vi "Process.vi"(8 "error in (no error)":errorcluster, 9 "Sensor Groups (false)":bool, 10 "Pound in":refnum<class "Pound.lvclass">, 11 "Qbus in":refnum<class "Qbus.lvclass">) -> (0 "error out":errorcluster)   [LabVIEW 2017, in "OPCUAClient.lvlib"]
uses:
  <vilib>/addons/InsightCM/Devices/Shared/Common/OPCUAClient/OPCUAClient.lvlib
  <vilib>/addons/Qbus/Qbus.lvclass
  <vilib>/NI/Software Watchdog/Pound/Pound.lvclass
  <vilib>/addons/InsightCM/Devices/Shared/Common/OPCUAClient/controls/config.ctl
  <vilib>/OPCUA/controls/OPC UA Client Refnum.ctl
  <vilib>/addons/InsightCM/Devices/Shared/Common/OPCUAClient/controls/group.ctl
  <vilib>/addons/InsightCM/Devices/Shared/Common/OPCUAClient/controls/tag.ctl
  <vilib>/OPCUA/controls/Time Out.ctl
  <vilib>/addons/TraceLogger/TraceLogger.lvlib
  <vilib>/NI/Software Watchdog/Watchdog/Watchdog.lvclass
  <vilib>/addons/InsightCM/Utilities/GlobalConfiguration/GlobalConfiguration.lvlib
  <vilib>/addons/InsightCM/Devices/Shared/Common/DataEventCreator/DataEventCreator.lvlib
  <vilib>/OPCUA/NI OPC UA Client.lvlib
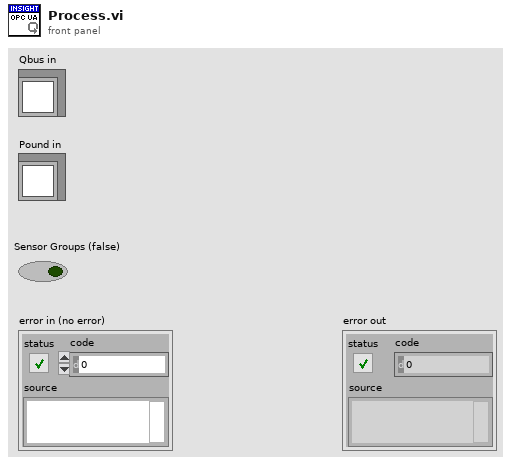
[diagram p1: front panel]
types:
  T1 = typedef "OPCUAClient.lvlib/config.ctl" = cluster{"OPC UA client refnum":T2, "Endpoint URL":string, "Client Certificate":path, "Server Certificate":path, "security policy":cluster{"message mode":enum16{"None", "Sign", "Sign and Encrypt"}, "security":enum16{"Basic256", "Basic128Rsa15"}}, "username/password":cluster{"username":string, "password":string}, "groups":T3[], "Read Interval (sec)":dbl, "Read Timeout (sec)":dbl, "Reconnect Interval (sec)":dbl, "Connection Timeout (sec)":dbl}
  T2 = typedef "OPC UA Client Refnum.ctl" = refnum<k21>
  T3 = typedef "OPCUAClient.lvlib/group.ctl" = cluster{"name":string, "Tags":T4[]}
  T4 = typedef "OPCUAClient.lvlib/tag.ctl" = cluster{"Id":string, "Tag":string, "Slope":dbl, "Offset":dbl}
  T5 = typedef "Time Out.ctl" = u32
  T6 = typedef "DataEventCreator.lvlib/RegisterTrendPoints.ctl" = cluster{"DataGroup":string, "Trends":T7[]}
  T7 = typedef "DataEventCreator.lvlib/Registry_Trend.ctl" = cluster{"TrendPointId":string, "DataSetName":string, "HighRate":bool, "Always Send":bool}
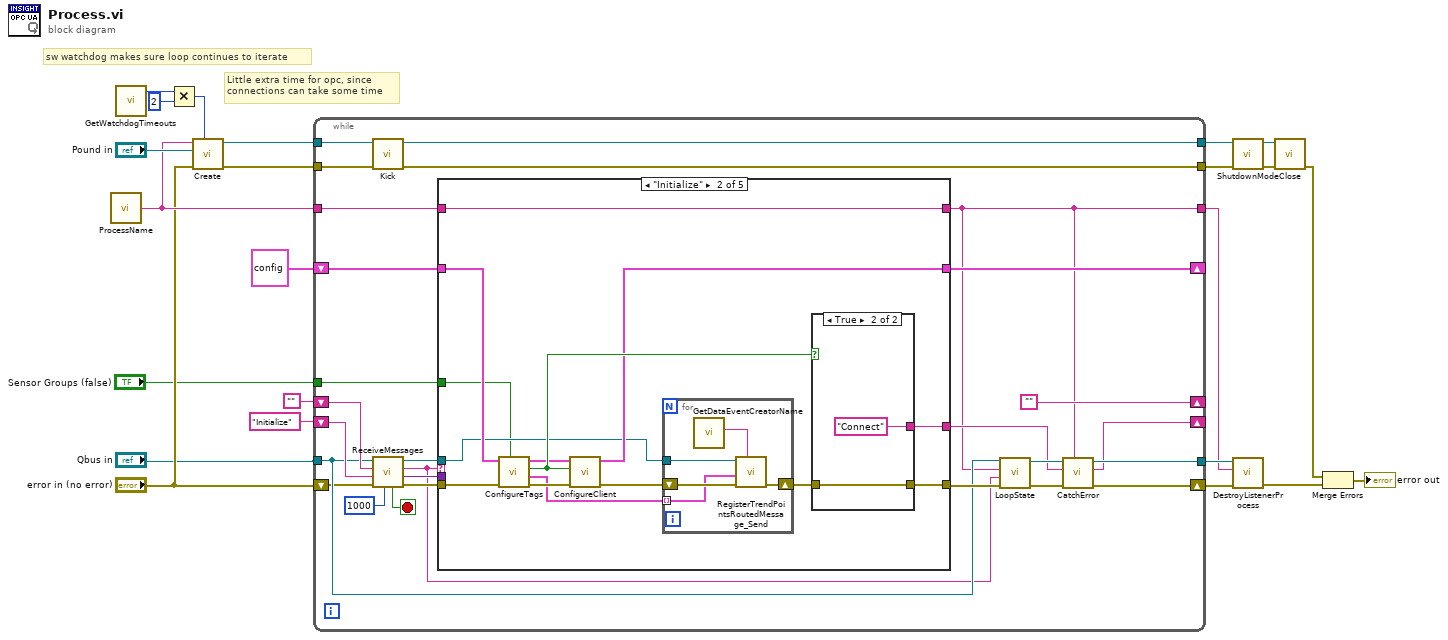
[diagram p0: block diagram]
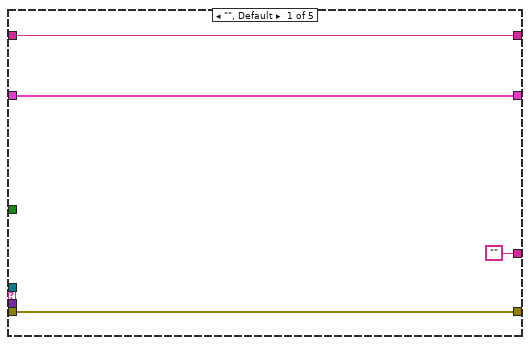
[diagram p2: hidden frame]
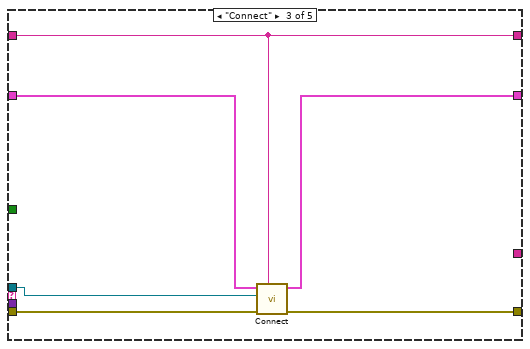
[diagram p4: hidden frame]
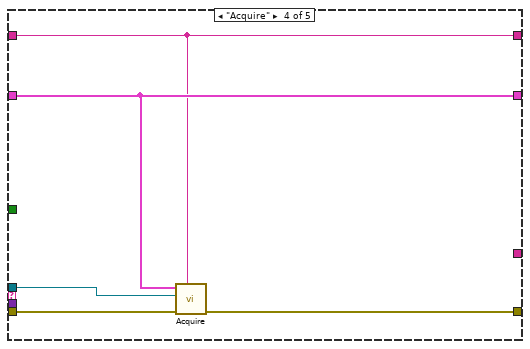
[diagram p5: hidden frame]
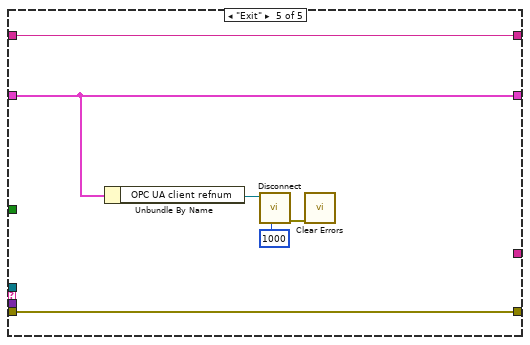
[diagram p6: hidden frame]
diagram:
  # "Little extra time for opc, since \nconnections can take some time"
  # "sw watchdog makes sure loop continues to iterate"
  n1 = call <vilib>:"ProcessName.vi"() -> ("process name"=w8:string)  [unwired: 5 in]
  n2 = call <vilib>:"GetWatchdogTimeouts.vi"() -> ("software timeout"=w3:u32)  [unwired: 10 in, 1 out]
  n3 = Multiply(x=w3, y=u32 2) -> (x*y=w1:u32)
  n4 = call <vilib>:"Create.vi"("Execution Timeout (ms)"=w1, "error in (no error)"="error in (no error)", "Pound"="Pound in", "Name"=w8) -> ("error out"=w13:errorcluster, "Watchdog"=w18:refnum<data-value>)  [unwired: 6 in]
  n5 = while {
    shift-right: [""] -> _
    shift-left: "" -> [w49]
    tunnel: "Qbus in" -> [w37]
    tunnel: w8 -> [w27]
    tunnel: [w40] -> w21
    tunnel: [w25] -> w20
    shift-right: [w39] -> _
    shift-left: "Initialize" -> [w44]
    shift-right: [w42] -> _
    shift-left: T1 {"OPC UA client refnum"="", "Endpoint URL"="", "Client Certificate"=path "", "Server Certificate"=path "", "security policy"={"message mode"=enum."None", "security"=enum."Basic256"}, "username/password"={"username"="", "password"=""}, "groups"=[], "Read Interval (sec)"=0.0, "Read Timeout (sec)"=0.0, "Reconnect Interval (sec)"=0.0, "Connection Timeout (sec)"=0.0} ("config") -> [w43]
    tunnel: w18 -> [w36]
    tunnel: [w35] -> w15
    tunnel: w13 -> [w34]
    tunnel: [w32] -> w12
    shift-right: [w41] -> w22
    shift-left: "error in (no error)" -> [w33]
    tunnel: "Sensor Groups (false)" -> [w24]
    stop <- w50 stop-if-true
    n6 = call <vilib>:"Kick.vi"("error in (no error)"=w34, "Watchdog"=w36) -> ("error out"=w32:errorcluster, "Watchdog"=w35:refnum<data-value>)  [unwired: 8 in]
    n7 = call <vilib>:"ReceiveMessages.vi"("Timeout(1000)"=1000 ("milliseconds to wait"), "error in (no error)"=w33, "priority action"=w44, "default action"=w49, "Qbus in"=w37) -> ("error out"=w48:errorcluster, "message value"=w45:variant, "action"=w31:string, "Qbus out"=w46:refnum<class "Qbus.lvclass">, "exit"=w50:bool)  [unwired: 2 in]
    n8 = case shown="\"Initialize\"" w31 {
      tunnel: w48 -> [w51 w64 w82 w86 w93]
      tunnel: w46 -> [_ w57 w78 w84 _]
      tunnel: [w51 w67 w77 w87 w93] -> w38
      tunnel: w45 -> [_ _ _ _ _]
      tunnel: w43 -> [w54 w65 w81 w85 w91]
      tunnel: [w54 w60 w80 w85 w91] -> w42
      tunnel: [w53 w68 w79 w83 w92] -> w25
      tunnel: w27 -> [w53 w68 w79 w83 w92]
      tunnel: ["" w66 _ _ _] -> w26
      tunnel: w24 -> [_ w55 _ _ _]
      frame "", Default {
      }
      frame "Initialize" {
        n9 = call <vilib>:"ConfigureTags.vi"("Sensor Groups (false)"=w55, "error in (no error)"=w64, "config in"=w65) -> ("error out"=w63:errorcluster, "Registrations"=w56:T6[], "Start OPC Client"=w62:bool, "config out"=w61:T1)  [unwired: 5 in]
        n10 = call <vilib>:"ConfigureClient.vi"("error in (no error)"=w63, "Start OPC Client"=w62, "config in"=w61) -> ("error out"=w59:errorcluster, "config out"=w60:T1)  [unwired: 7 in]
        n11 = for {
          shift-right: [w72] -> w58
          shift-left: w59 -> [w73]
          tunnel: w57 -> [w71]
          tunnel: w56 -> [w70] mode=indexing
          n12 = call <vilib>:"GetDataEventCreatorName.vi"() -> ("data event creator"=w69:string)  [unwired: 9 in, 2 out]
          n13 = call <vilib>:"RegisterTrendPointsRoutedMessage_Send.vi"("data event creator process name"=w69, "error in (no error)"=w73, "register trend"=w70, "Qbus in"=w71) -> ("error out"=w72:errorcluster)  [unwired: 6 in, 1 out]
        }
        n14 = case shown="True" w62 {
          tunnel: [w74 w76] -> w67
          tunnel: w58 -> [w74 w76]
          tunnel: [_ "Connect"] -> w66
          frame False {
          }
          frame True {
          }
        }
      }
      frame "Connect" {
        n15 = call <vilib>:"Connect.vi"("Process Name"=w79, "error in (no error)"=w82, "Qbus"=w78, "config"=w81) -> ("error out"=w77:errorcluster, "config out"=w80:T1)  [unwired: 5 in, 1 out]
      }
      frame "Acquire" {
        n16 = call <vilib>:"Acquire.vi"("Module Name"=w83, "error in (no error)"=w86, "Qbus in"=w84, "config"=w85) -> ("error out"=w87:errorcluster)  [unwired: 7 in]
      }
      frame "Exit" {
        n17 = Unbundle By Name(w91) -> ("OPC UA client refnum"=w90:T2)
        n18 = call <vilib>:"Disconnect.vi"("timeout (5000 ms)"=T5 1000, "OPC UA client refnum in"=w90) -> ("error out"=w89:errorcluster)  [unwired: 9 in]
        n19 = call <vilib>:"Clear Errors.vi"("error in (no error)"=w89) -> ()  [unwired: 5 in, 2 out]
      }
    }
    n20 = call <vilib>:"LoopState.vi"("error in (no error)"=w38, "loop action"=w31, "process name"=w25, "Qbus in"=w37) -> ("error out"=w29:errorcluster, "Qbus out"=w28:refnum<class "Qbus.lvclass">)  [unwired: 6 in]
    n21 = call <vilib>:"CatchError.vi"("source"=w25, "error in (no error)"=w29, "next action in"=w26, "Qbus in"=w28) -> ("error out"=w41:errorcluster, "next action out"=w39:string, "Qbus out"=w40:refnum<class "Qbus.lvclass">)  [unwired: 5 in]
  }
  n22 = call <vilib>:"ShutdownMode.vi"("error in (no error)"=w12, "Watchdog"=w15) -> ("error out"=w14:errorcluster, "Watchdog"=w16:refnum<data-value>)  [unwired: 8 in]
  n23 = call <vilib>:"DestroyListenerProcess.vi"("error in (no error)"=w22, "process name"=w20, "Qbus in"=w21) -> ("error in (no error)"=w11:errorcluster)  [unwired: 7 in, 1 out]
  n24 = call <vilib>:"Close.vi"("error in (no error)"=w14, "Watchdog"=w16) -> ("error out"=w10:errorcluster)  [unwired: 9 in]
  n25 = Merge Errors(w10, w11) -> (→"error out":errorcluster)
